vi "17_SoftwareClock.vi"(8 "error in (no error)":errorcluster) -> (0 "error out":errorcluster)   [LabVIEW 2014]
uses:
  SwabianInstruments.TimeTagger
panel:
  out "SoftwareClockState":T1={"enabled"=FALSE, "is_locked"=FALSE, "period_error"=nan, "phase_error_estimation"=nan, "clock_period"=0, "error_counter"=0}
  in  "SoftwareClock settings":T2={"clock source"=enum."test signal as external clock", "input freq."=900000.0, "averaging_periods"=100.0, "trace_len"=1000, "clock channel"=1}
  in  "FrequencyStability settings":T3={"average"=1, "steps start"=1, "steps end"=100000, "number of steps"=100, "signal source"=enum."test signal", "signal channel"=2} {"number of steps" min=2 max=1000}
  out "Frequency error":T4(graph)
  out "Phase error":T5(graph)
  out "logger output":string="########################\n\nThis example demonstrates the SoftwareClock. The SoftwareClock is the recommended way to apply an external clock to the Time Tagger. Here, we will use the internal test signal for demonstration purposes. Be aware that this means decreasing the quality of the internal clock of your Time Tagger! If you have a high-quality external reference available, feel free to apply this and to set \"clock source\" to \"external clock\".\n\nThe settings of the SoftwareClock are updated every when the measurement is started.\n\nThe FrequencyStability measurement class provides numerous standard metrics conforming to IEEE 1139, e.g. the Allan Deviation (ADEV).\n\n########################\r\n\r\n"
  in  "exit":bool
  in  "run measurement":bool
  out "Time domain":cluster{"getTau":dbl[], "getHDEV":dbl[]}[](graph)
  out "Allan domain":cluster{"getTau":dbl[], "getSTDD":dbl[]}[](graph)
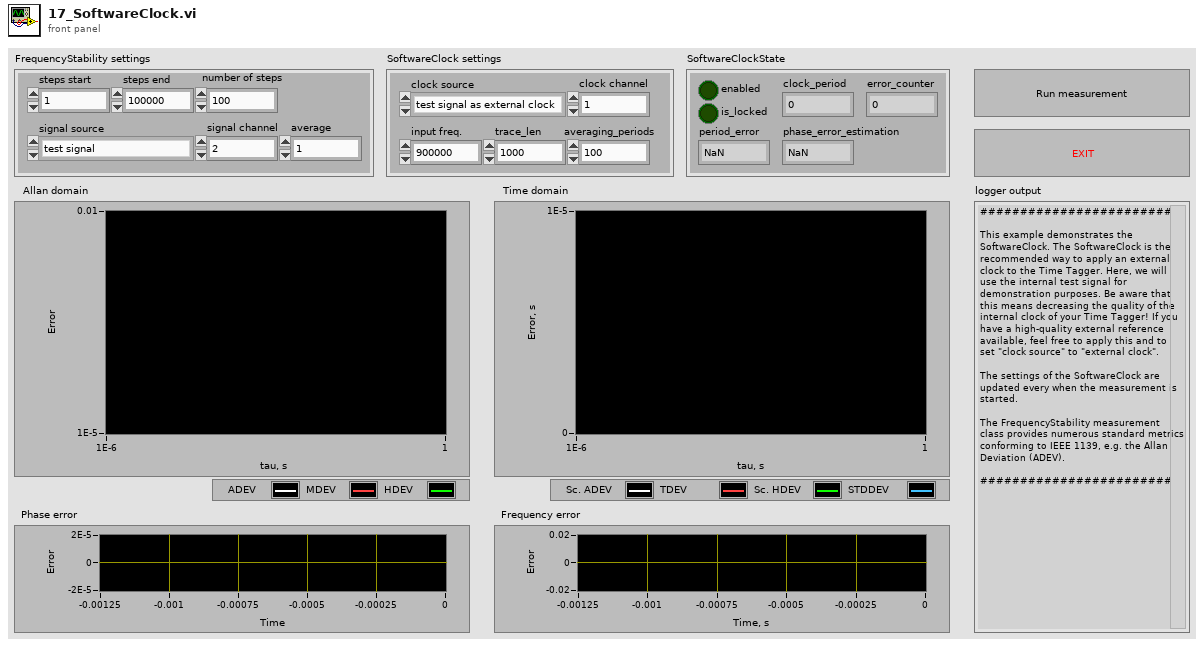
[diagram p1: front panel]
types:
  T1 = cluster{"enabled":bool, "is_locked":bool, "period_error":dbl, "phase_error_estimation":dbl, "clock_period":i64, "error_counter":i64}
  T2 = cluster{"clock source":enum16{"internal clock", "external clock", "test signal as external clock"}, "input freq.":dbl, "averaging_periods":dbl, "trace_len":u64, "clock channel":i32}
  T3 = cluster{"average":i64, "steps start":i32, "steps end":i32, "number of steps":i32, "signal source":enum16{"external signal", "test signal"}, "signal channel":i32}
  T4 = cluster{"getTraceIndex":dbl[], "getTraceFrequency":dbl[]}
  T5 = cluster{"getTraceIndex":dbl[], "getTracePhase":dbl[]}
  T6 = enum16{"internal clock", "external clock", "test signal as external clock"}
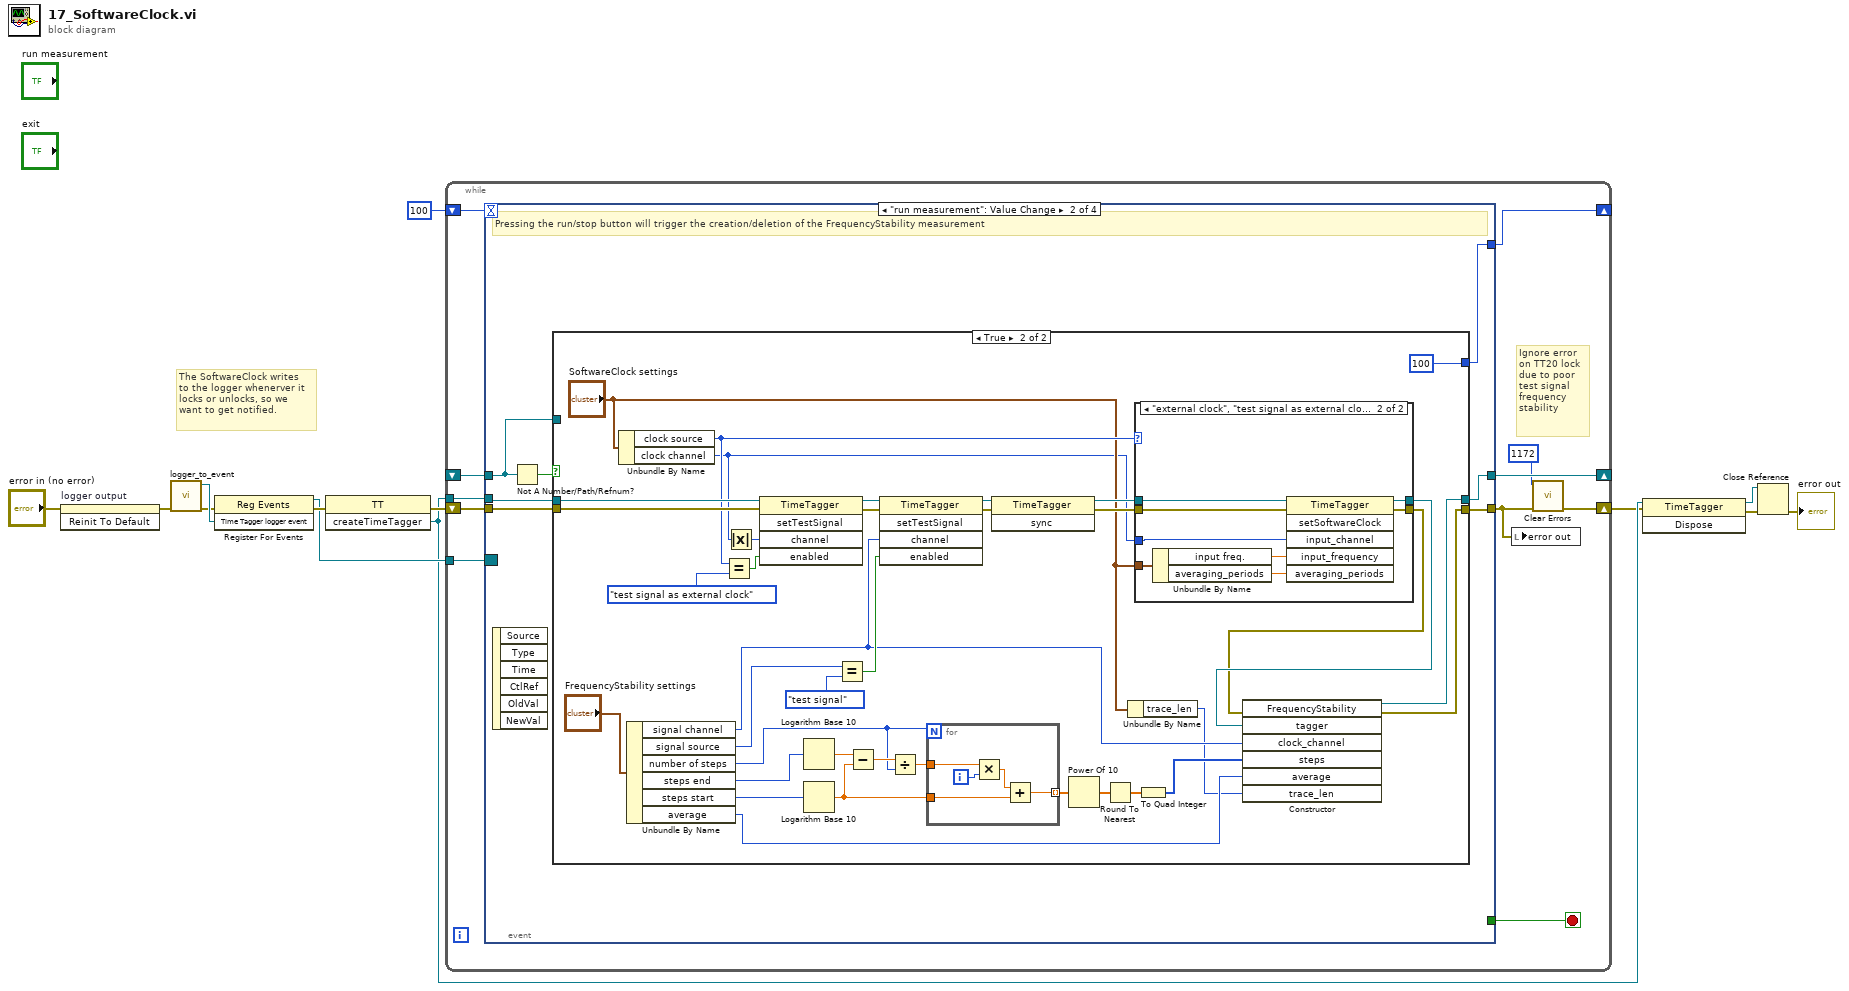
[diagram p0: block diagram]
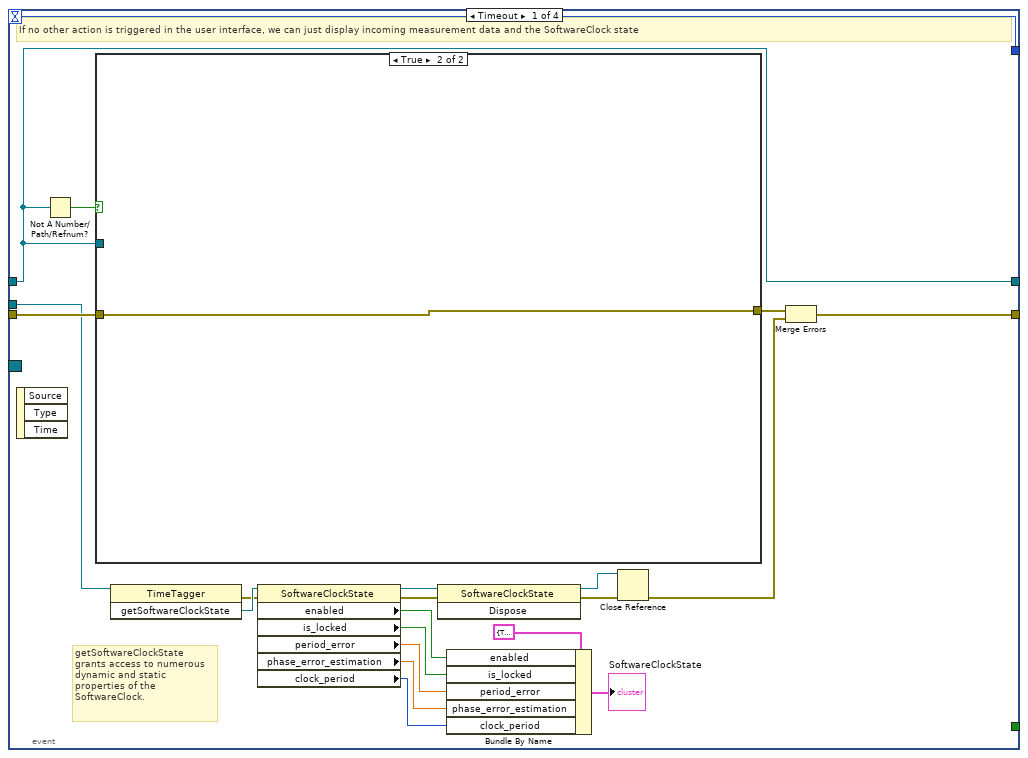
[diagram p2: hidden frame]
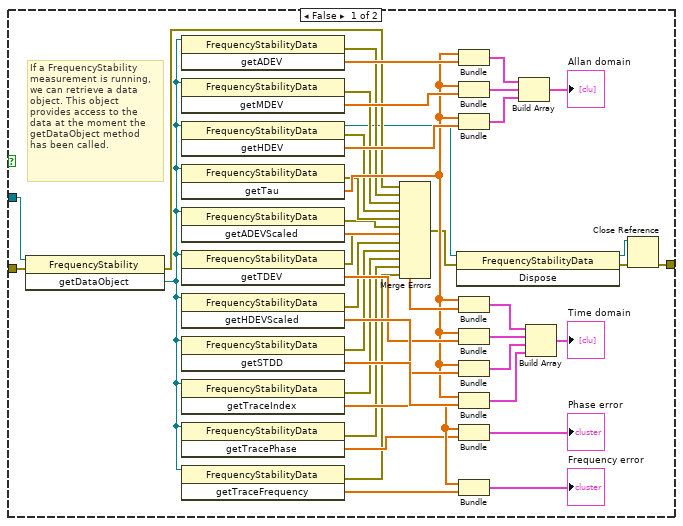
[diagram p3: hidden frame]
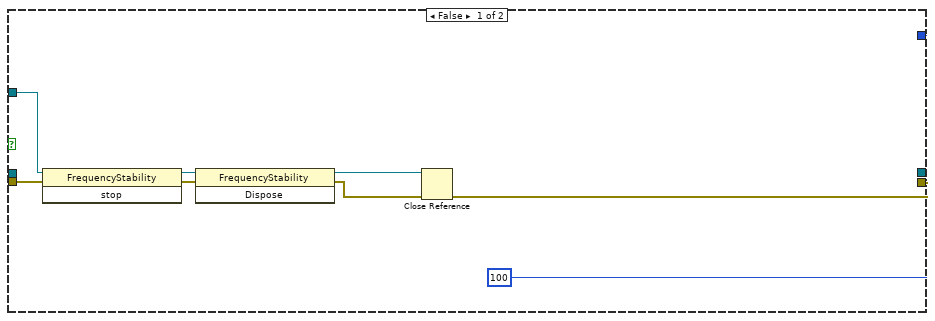
[diagram p4: hidden frame]
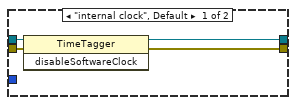
[diagram p5: hidden frame]
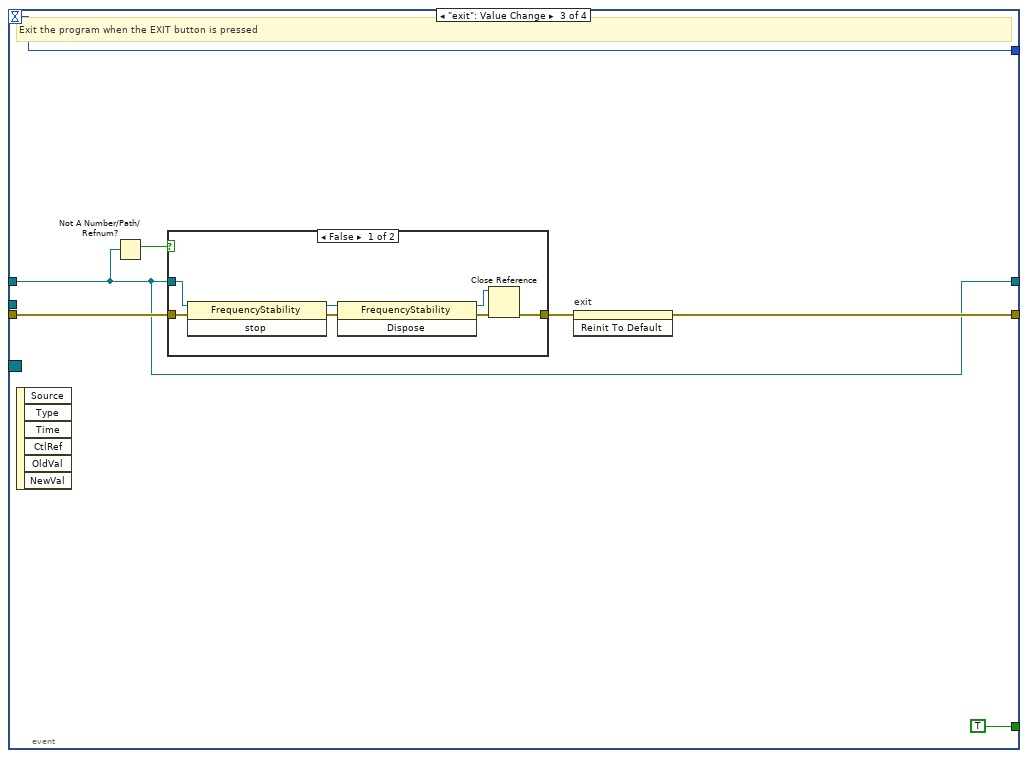
[diagram p6: hidden frame]
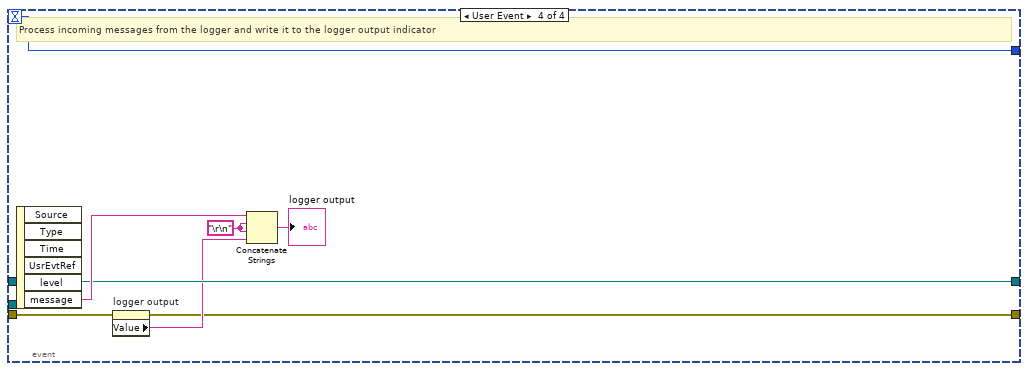
[diagram p8: hidden frame]
diagram:
  # "The SoftwareClock writes\nto the logger whenerver it\nlocks or unlocks, so we\nwant to get notified."
  n1 = invoke on="logger output" class="Str" method="Reinit To Default"(error in="error in (no error)") -> (error out=w7:errorcluster)  [unwired: 2 in, 2 out]
  n2 = call "logger_to_event.vi"("error in (no error)"=w7) -> ("error out"=w10:errorcluster, "Time Tagger logger event"=w11:refnum<user-event>)  [unwired: 9 in]
  n3 = register-events(error in=w10, w11) -> (reference out=w8:refnum<event-registration>, error out=w9:errorcluster)  [unwired: 1 in]
  n4 = invoke class="TT" method="createTimeTagger"(error in=w9) -> (error out=w12:errorcluster, "createTimeTagger"=w6:refnum<k24>)  [unwired: 2 in, 1 out]
  n5 = while {
    tunnel: w6 -> [w24]
    shift-right: [w23] -> _
    shift-left: _ -> [w22]
    shift-right: [w20] -> _
    shift-left: 100 -> [w21]
    shift-right: [w16] -> w1
    shift-left: w12 -> [w19]
    tunnel: w8 -> [w17]
    stop <- w18 stop-if-true
    # "Ignore error\non TT20 lock \ndue to poor\ntest signal\nfrequency \nstability"
    n6 = event shown="[1] \"run measurement\": Value Change" {
      selector: w17 -> [_ _ _ _]
      dyn-events: _ -> [_ _ _ _]
      timeout: w21 -> [w28 _ w162 w178]
      tunnel: w24 -> [w43 w95 _ _]
      tunnel: [w45 w94 w158 w179] -> w23
      tunnel: w22 -> [w45 w92 w158 w179]
      tunnel: [w28 w91 w162 w178] -> w20
      tunnel: w19 -> [w44 w90 w159 w173]
      tunnel: [w26 w89 w164 w174] -> w15
      tunnel: [_ _ TRUE _] -> w18
      event Timeout {
        # "getSoftwareClockState\ngrants access to numerous\ndynamic and static\nproperties of the\nSoftwareClock."
        # "If no other action is triggered in the user interface, we can just display incoming measurement data and the SoftwareClock state"
        n7 = event-data() -> ()  [unwired: 1 in, 3 out]
        n8 = Not A Number/Path/Refnum?(number/path/refnum=w45) -> (NaN/Path/Refnum?=w42:bool)
        n9 = case shown="True" w42 {
          tunnel: w45 -> [w87 _]
          tunnel: w44 -> [w86 w88]
          tunnel: [w64 w88] -> w27
          frame False {
            # "If a FrequencyStability\nmeasurement is running,\nwe can retrieve a data\nobject. This object\nprovides access to the\ndata at the moment the\ngetDataObject method\nhas been called."
            n10 = invoke class="FrequencyStability" method="getDataObject"(reference=w87, error in=w86) -> (error out=w68:errorcluster, "getDataObject"=w63:refnum<k24>)  [unwired: 1 in, 1 out]
            n11 = invoke class="FrequencyStabilityData" method="getADEV"(reference=w63) -> (error out=w57:errorcluster, "getADEV"=w85:dbl[])  [unwired: 2 in, 1 out]
            n12 = invoke class="FrequencyStabilityData" method="getMDEV"(reference=w63) -> (error out=w56:errorcluster, "getMDEV"=w84:dbl[])  [unwired: 2 in, 1 out]
            n13 = invoke class="FrequencyStabilityData" method="getHDEV"(reference=w63) -> (reference out=w46:refnum<k24>, error out=w55:errorcluster, "getHDEV"=w83:dbl[])  [unwired: 2 in]
            n14 = invoke class="FrequencyStabilityData" method="getTau"(reference=w63) -> (error out=w54:errorcluster, "getTau"=w78:dbl[])  [unwired: 2 in, 1 out]
            n15 = invoke class="FrequencyStabilityData" method="getADEVScaled"(reference=w63) -> (error out=w53:errorcluster, "getADEVScaled"=w79:dbl[])  [unwired: 2 in, 1 out]
            n16 = invoke class="FrequencyStabilityData" method="getTDEV"(reference=w63) -> (error out=w52:errorcluster, "getTDEV"=w80:dbl[])  [unwired: 2 in, 1 out]
            n17 = invoke class="FrequencyStabilityData" method="getHDEVScaled"(reference=w63) -> (error out=w51:errorcluster, "getHDEVScaled"=w81:dbl[])  [unwired: 2 in, 1 out]
            n18 = invoke class="FrequencyStabilityData" method="getSTDD"(reference=w63) -> (error out=w50:errorcluster, "getSTDD"=w82:dbl[])  [unwired: 2 in, 1 out]
            n19 = invoke class="FrequencyStabilityData" method="getTraceIndex"(reference=w63) -> (error out=w49:errorcluster, "getTraceIndex"=w61:dbl[])  [unwired: 2 in, 1 out]
            n20 = invoke class="FrequencyStabilityData" method="getTracePhase"(reference=w63) -> (error out=w48:errorcluster, "getTracePhase"=w60:dbl[])  [unwired: 2 in, 1 out]
            n21 = invoke class="FrequencyStabilityData" method="getTraceFrequency"(reference=w63) -> (error out=w47:errorcluster, "getTraceFrequency"=w62:dbl[])  [unwired: 2 in, 1 out]
            n22 = Merge Errors(w68, w57, w56, w55, w54, w53, w52, w51, w50, w49, w48, w47) -> (w67:errorcluster)
            n23 = invoke class="FrequencyStabilityData" method="Dispose"(reference=w46, error in=w67) -> (reference out=w66:refnum<k24>, error out=w65:errorcluster)  [unwired: 1 in, 1 out]
            n24 = Bundle("getTau"=w78, "getADEV"=w85) -> (w77:cluster{"getTau":dbl[], "getADEV":dbl[]})  [unwired: 1 in]
            n25 = Bundle("getTau"=w78, "getMDEV"=w84) -> (w76:cluster{"getTau":dbl[], "getMDEV":dbl[]})  [unwired: 1 in]
            n26 = Bundle("getTau"=w78, "getHDEV"=w83) -> (w75:cluster{"getTau":dbl[], "getHDEV":dbl[]})  [unwired: 1 in]
            n27 = Bundle("getTau"=w78, "getADEVScaled"=w79) -> (w74:cluster{"getTau":dbl[], "getADEVScaled":dbl[]})  [unwired: 1 in]
            n28 = Bundle("getTau"=w78, "getTDEV"=w80) -> (w73:cluster{"getTau":dbl[], "getTDEV":dbl[]})  [unwired: 1 in]
            n29 = Bundle("getTau"=w78, "getHDEVScaled"=w81) -> (w72:cluster{"getTau":dbl[], "getHDEVScaled":dbl[]})  [unwired: 1 in]
            n30 = Bundle("getTau"=w78, "getSTDD"=w82) -> (w71:cluster{"getTau":dbl[], "getSTDD":dbl[]})  [unwired: 1 in]
            n31 = Bundle("getTraceIndex"=w61, "getTracePhase"=w60) -> (→"Phase error":T5)  [unwired: 1 in]
            n32 = Bundle("getTraceIndex"=w61, "getTraceFrequency"=w62) -> (→"Frequency error":T4)  [unwired: 1 in]
            n33 = Build Array(w77, w76, w75) -> (→"Allan domain":cluster{"getTau":dbl[], "getHDEV":dbl[]}[])
            n34 = Build Array(w74, w73, w72, w71) -> (→"Time domain":cluster{"getTau":dbl[], "getSTDD":dbl[]}[])
            n35 = Close Reference(reference=w66, error in (no error)=w65) -> (error out=w64:errorcluster)
          }
          frame True {
          }
        }
        n36 = invoke class="TimeTagger" method="getSoftwareClockState"(reference=w43) -> (error out=w40:errorcluster, "getSoftwareClockState"=w41:refnum<k24>)  [unwired: 2 in, 1 out]
        n37 = property class="SoftwareClockState"(reference=w41, error in=w40) -> (reference out=w30:refnum<k24>, error out=w31:errorcluster, "enabled"=w39:bool, "is_locked"=w38:bool, "period_error"=w37:dbl, "phase_error_estimation"=w35:dbl, "clock_period"=w34:i64)
        n38 = invoke class="SoftwareClockState" method="Dispose"(reference=w30, error in=w31) -> (reference out=w33:refnum<k24>, error out=w32:errorcluster)  [unwired: 1 in, 1 out]
        n39 = Bundle By Name(cluster=T1 {"enabled"=TRUE, "is_locked"=TRUE, "period_error"=34575.234590264736, "phase_error_estimation"=8484.866795079515, "clock_period"=1111111, "error_counter"=1111111} ("SoftwareClockState"), "enabled"=w39, "is_locked"=w38, "period_error"=w37, "phase_error_estimation"=w35, "clock_period"=w34) -> (→"SoftwareClockState":T1)
        n40 = Close Reference(reference=w33, error in (no error)=w32) -> (error out=w25:errorcluster)
        n41 = Merge Errors(w27, w25) -> (w26:errorcluster)
      }
      event "run measurement": Value Change {
        # "Pressing the run/stop button will trigger the creation/deletion of the FrequencyStability measurement"
        n42 = event-data() -> ()  [unwired: 1 in, 6 out]
        n43 = Not A Number/Path/Refnum?(number/path/refnum=w92) -> (NaN/Path/Refnum?=w93:bool)
        n44 = case shown="True" w93 {
          tunnel: w95 -> [_ w119]
          tunnel: [_ w140] -> w94
          tunnel: w92 -> [w102 _]
          tunnel: [100 100] -> w91
          tunnel: w90 -> [w101 w132]
          tunnel: [w96 w127] -> w89
          frame False {
            n45 = invoke class="FrequencyStability" method="stop"(reference=w102, error in=w101) -> (reference out=w100:refnum<k24>, error out=w99:errorcluster)  [unwired: 1 in, 1 out]
            n46 = invoke class="FrequencyStability" method="Dispose"(reference=w100, error in=w99) -> (reference out=w98:refnum<k24>, error out=w97:errorcluster)  [unwired: 1 in, 1 out]
            n47 = Close Reference(reference=w98, error in (no error)=w97) -> (error out=w96:errorcluster)
          }
          frame True {
            n48 = Unbundle By Name("SoftwareClock settings") -> ("clock source"=w113:T6, "clock channel"=w109:i32)
            n49 = Unbundle By Name("FrequencyStability settings") -> ("signal channel"=w108:i32, "signal source"=w112:enum16{"external signal", "test signal"}, "number of steps"=w104:i32, "steps end"=w107:i32, "steps start"=w116:i32, "average"=w117:i64)
            n50 = Equal?(x=w113, y=T6."test signal as external clock") -> (x = y?=w114:bool)
            n51 = Absolute Value(x=w109) -> (abs(x)=w115:i32)
            n52 = invoke class="TimeTagger" method="setTestSignal"(reference=w119, error in=w132, "channel"=w115, "enabled"=w114) -> (reference out=w130:refnum<k24>, error out=w131:errorcluster)  [unwired: 1 in, 3 out]
            n53 = Logarithm Base 10(1:w107) -> (0:w137:dbl)
            n54 = Logarithm Base 10(1:w116) -> (0:w105:dbl)
            n55 = Equal?(x=w112, y=enum16{"external signal", "test signal"}."test signal") -> (x = y?=w121:bool)
            n56 = Subtract(x=w137, y=w105) -> (x-y=w139:dbl)
            n57 = invoke class="TimeTagger" method="setTestSignal"(reference=w130, error in=w131, "channel"=w108, "enabled"=w121) -> (reference out=w126:refnum<k24>, error out=w124:errorcluster)  [unwired: 1 in, 3 out]
            n58 = Divide(x=w139, y=w104) -> (x/y=w138:dbl)
            n59 = for {
              N: w104 -> [_]
              tunnel: w138 -> [w157]
              tunnel: [w154] -> w136 mode=indexing
              tunnel: w105 -> [w153]
              i -> [w156]
              n60 = Multiply(x=w157, y=w156) -> (x*y=w155:dbl)
              n61 = Add(x=w155, y=w153) -> (x+y=w154:dbl)
            }
            n62 = invoke class="TimeTagger" method="sync"(reference=w126, error in=w124) -> (reference out=w125:refnum<k24>, error out=w123:errorcluster)  [unwired: 1 in, 1 out]
            n63 = Power Of 10(x=w136) -> (10^x=w135:dbl[])
            n64 = Round To Nearest(number=w135) -> (nearest integer value=w134:dbl[])
            n65 = Unbundle By Name("SoftwareClock settings") -> ("trace_len"=w106:u64)
            n66 = case shown="\"external clock\", \"test signal as external clock\"" w113 {
              tunnel: [w141 w152] -> w129
              tunnel: [w142 w151] -> w128
              tunnel: w109 -> [_ w150]
              tunnel: w125 -> [w144 w149]
              tunnel: w123 -> [w143 w148]
              tunnel: "SoftwareClock settings" -> [_ w147]
              frame "internal clock", Default {
                n67 = invoke class="TimeTagger" method="disableSoftwareClock"(reference=w144, error in=w143) -> (reference out=w141:refnum<k24>, error out=w142:errorcluster)  [unwired: 1 in, 1 out]
              }
              frame "external clock", "test signal as external clock" {
                n68 = Unbundle By Name(w147) -> ("input freq."=w146:dbl, "averaging_periods"=w145:dbl)
                n69 = invoke class="TimeTagger" method="setSoftwareClock"(reference=w149, error in=w148, "input_channel"=w150, "input_frequency"=w146, "averaging_periods"=w145) -> (reference out=w152:refnum<k24>, error out=w151:errorcluster)  [unwired: 1 in, 4 out]
              }
            }
            n70 = To Quad Integer(1:w134) -> (0:w133:i64[])
            n71 = constructor class="FrequencyStability"(error in=w128, "tagger"=w129, "clock_channel"=w108, "steps"=w133, "average"=w117, "trace_len"=w106) -> (reference out=w140:refnum<k24>, error out=w127:errorcluster)  [unwired: 2 in, 6 out]
          }
        }
      }
      event "exit": Value Change {
        # "Exit the program when the EXIT button is pressed"
        n72 = event-data() -> ()  [unwired: 1 in, 6 out]
        n73 = Not A Number/Path/Refnum?(number/path/refnum=w158) -> (NaN/Path/Refnum?=w161:bool)
        n74 = case shown="False" w161 {
          tunnel: w158 -> [w166 _]
          tunnel: [w167 w172] -> w160
          tunnel: w159 -> [w165 w172]
          frame False {
            n75 = invoke class="FrequencyStability" method="stop"(reference=w166, error in=w165) -> (reference out=w171:refnum<k24>, error out=w170:errorcluster)  [unwired: 1 in, 1 out]
            n76 = invoke class="FrequencyStability" method="Dispose"(reference=w171, error in=w170) -> (reference out=w169:refnum<k24>, error out=w168:errorcluster)  [unwired: 1 in, 1 out]
            n77 = Close Reference(reference=w169, error in (no error)=w168) -> (error out=w167:errorcluster)
          }
          frame True {
          }
        }
        n78 = invoke on="exit" class="Bool (strict)" method="Reinit To Default"(error in=w160) -> (error out=w164:errorcluster)  [unwired: 2 in, 2 out]
      }
      event User Event {
        w177 = "\r\n"
        # "Process incoming messages from the logger and write it to the logger output indicator"
        n79 = event-data() -> ("message"=w180:string)  [unwired: 1 in, 5 out]
        n80 = property on="logger output" class="Str"(error in=w173) -> (error out=w174:errorcluster, "Value"=w176:string)  [unwired: 1 in, 1 out]
        n81 = Concatenate Strings(w180, w177, w177, w176) -> (→"logger output":string)
      }
    }
    n82 = local write "error out"(w15) -> ()
    n83 = call <vilib>:"Clear Errors.vi"("error in (no error)"=w15, "specific error code to clear (0: all)"=1172) -> ("error out"=w16:errorcluster)  [unwired: 4 in, 1 out]
  }
  n84 = invoke class="TimeTagger" method="Dispose"(reference=w6, error in=w1) -> (reference out=w4:refnum<k24>, error out=w5:errorcluster)  [unwired: 1 in, 1 out]
  n85 = Close Reference(reference=w4, error in (no error)=w5) -> (error out=→"error out":errorcluster)
